vi "Calculadora_m.vi"() -> ()   [LabVIEW 2019]
panel:
  out "Alerta":string
  out "Resultado":dbl
  in  "Division":bool
  in  "Resta":bool
  in  "Multiplicacion":bool
  in  "Suma":bool
  in  "Numero 2":dbl
  in  "Numero 1":dbl
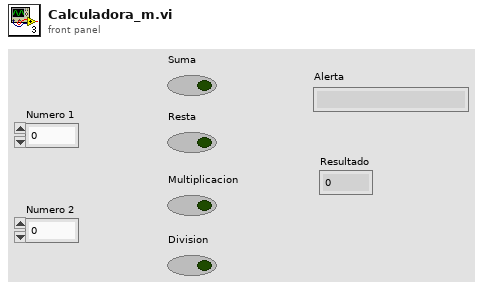
[diagram p1: front panel]
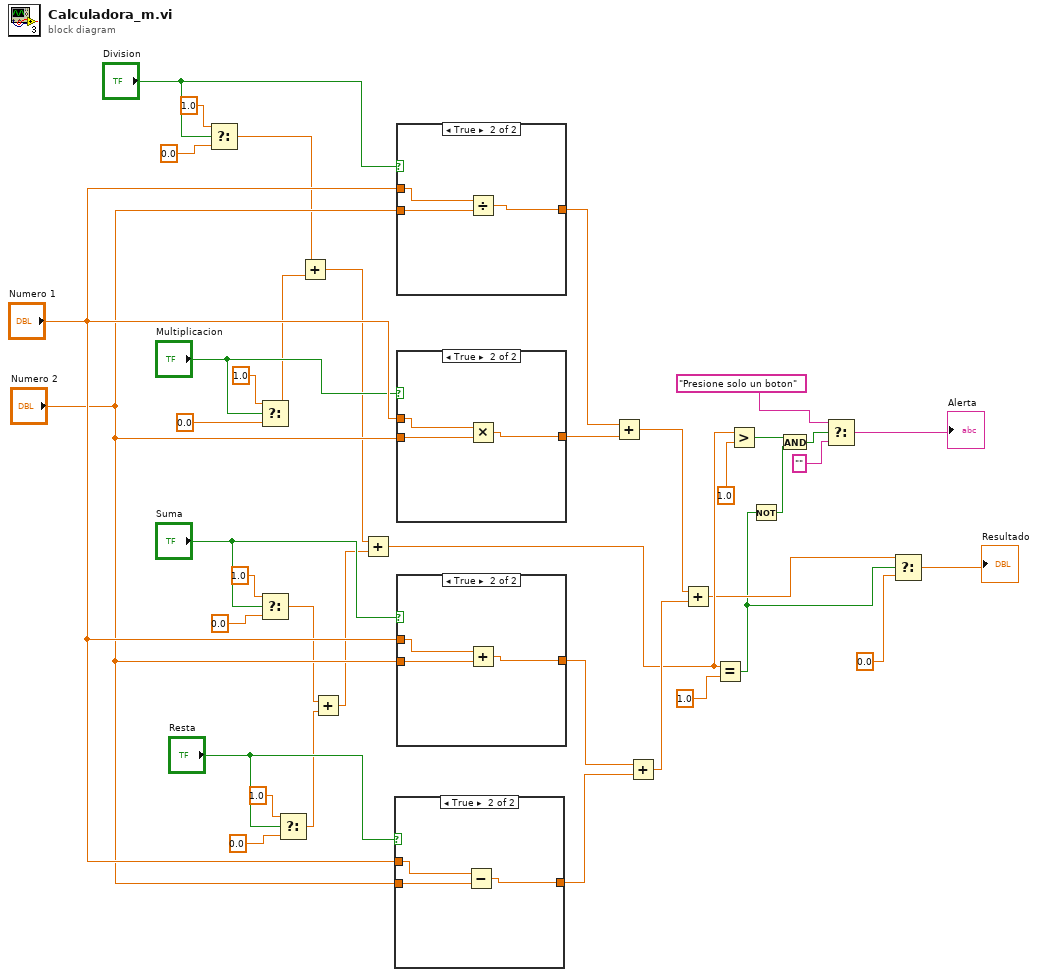
[diagram p0: block diagram]
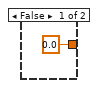
[diagram p2: hidden frame]
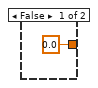
[diagram p3: hidden frame]
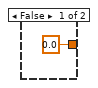
[diagram p4: hidden frame]
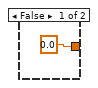
[diagram p5: hidden frame]
diagram:
  n1 = Select(t=1.0, s="Division", f=0.0) -> (s? t:f=w29:dbl)
  n2 = Select(t=1.0, s="Multiplicacion", f=0.0) -> (s? t:f=w25:dbl)
  n3 = Select(t=1.0, s="Suma", f=0.0) -> (s? t:f=w17:dbl)
  n4 = Select(t=1.0, s="Resta", f=0.0) -> (s? t:f=w18:dbl)
  n5 = Add(x=w29, y=w25) -> (x+y=w15:dbl)
  n6 = Add(x=w17, y=w18) -> (x+y=w16:dbl)
  n7 = Add(x=w15, y=w16) -> (x+y=w8:dbl)
  n8 = case shown="True" "Resta" {
    tunnel: "Numero 1" -> [_ w43]
    tunnel: "Numero 2" -> [_ w42]
    tunnel: [0.0 w41] -> w34
    frame False {
    }
    frame True {
      n9 = Subtract(x=w43, y=w42) -> (x-y=w41:dbl)
    }
  }
  n10 = case shown="True" "Division" {
    tunnel: "Numero 1" -> [_ w47]
    tunnel: "Numero 2" -> [_ w46]
    tunnel: [0.0 w45] -> w38
    frame False {
    }
    frame True {
      n11 = Divide(x=w47, y=w46) -> (x/y=w45:dbl)
    }
  }
  n12 = case shown="True" "Multiplicacion" {
    tunnel: "Numero 1" -> [_ w51]
    tunnel: "Numero 2" -> [_ w50]
    tunnel: [0.0 w49] -> w39
    frame False {
    }
    frame True {
      n13 = Multiply(x=w51, y=w50) -> (x*y=w49:dbl)
    }
  }
  n14 = case shown="True" "Suma" {
    tunnel: "Numero 1" -> [_ w55]
    tunnel: "Numero 2" -> [_ w54]
    tunnel: [0.0 w53] -> w35
    frame False {
    }
    frame True {
      n15 = Add(x=w55, y=w54) -> (x+y=w53:dbl)
    }
  }
  n16 = Add(x=w38, y=w39) -> (x+y=w13:dbl)
  n17 = Add(x=w35, y=w34) -> (x+y=w33:dbl)
  n18 = Add(x=w13, y=w33) -> (x+y=w4:dbl)
  n19 = Equal?(x=w8, y=1.0) -> (x = y?=w3:bool)
  n20 = Greater?(x=w8, y=1.0) -> (0:w9:bool)
  n21 = Not(x=w3) -> (.not. x?=w6:bool)
  n22 = And(x=w9, y=w6) -> (x .and. y?=w5:bool)
  n23 = Select(t="Presione solo un boton", s=w5, f="") -> (s? t:f=→"Alerta":string)
  n24 = Select(t=w4, s=w3, f=0.0) -> (s? t:f=→"Resultado":dbl)
